vi "Write File Path.vi"(8 "error in (no error)":errorcluster, 10 "File Ref":refnum<file>, 11 "Read in":refnum<class "Read.lvclass">) -> (0 "error out":errorcluster, 3 "Read out":refnum<class "Read.lvclass">)   [LabVIEW 2014, in "Read.lvclass"]
uses:
  Read.lvclass
  Read.lvclass/Read.ctl
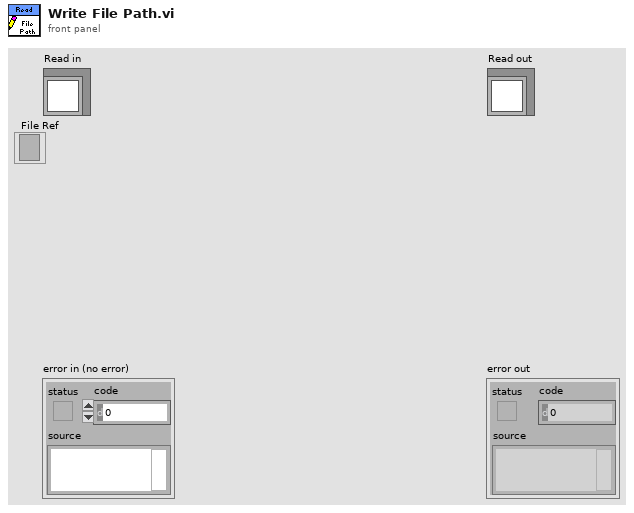
[diagram p1: front panel]
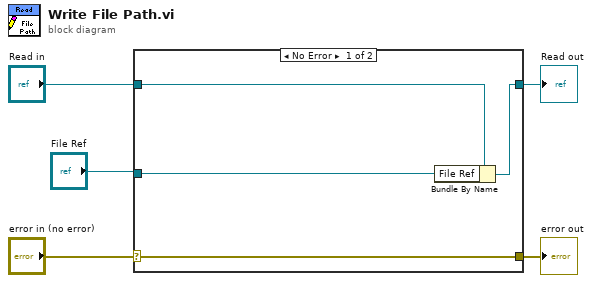
[diagram p0: block diagram]
diagram:
  n1 = case shown="No Error" "error in (no error)" {
    selector: "error in (no error)" -> [w9 w10]
    tunnel: [w9 w10] -> w4
    tunnel: [w7 w11] -> w2
    tunnel: "Read in" -> [w8 w11]
    tunnel: "File Ref" -> [w6 _]
    frame No Error {
      n2 = Bundle By Name(cluster=w8, "File Ref"=w6) -> (w7:refnum<class "Read.lvclass">)
    }
    frame Error {
    }
  }
  "error out" <- w4
  "Read out" <- w2
